vi "Get Cluster Element Names.vi"(8 "error in (no error)":errorcluster, 10 "Cluster":variant) -> (0 "error out":errorcluster, 2 "Element Names":string[](array[string]))   [LabVIEW 2020]
doc: "Returns the data names of the cluster elements."
panel:
  # "[OpenG VI Tags] ***Do Not Remove***"
  # "Get Cluster Element Names.vi\n\nReturns the data names of the cluster elements.\n\nPlease visit http://www.OpenG.org to learn about the\nOpen Source LabVIEW software movement.\n\nNOTICE -- YOU MUST LEAVE THIS NOTICE IN PLACE.  PER THE TERMS OF THE LICENSE BELOW, YOU MAY SUBLICENSE THIS SOFTWARE \nIN ANY WAY THAT DOES NOT CONFLICT WITH THIS LICENSE.\n\n### BSD License (http://www.opensource.org/licenses/bsd-license.php) Begin ###\n \nCopyright (c) 2002, Jean-Pierre Drolet <drolet_jp@hotmail.com>\nCopyright (c) 2002-2006, Jim Kring <jim@jimkring.com>\n\nAll rights reserved.\n\nRedistribution and use in source and binary forms, with or without modification, are permitted provided that the following conditions are met:\n\n    * Redistributions of source code must retain the above copyright notice, this list of conditions and the following disclaimer.\n    * Redistributions in binary form must reproduce the above copyright notice, this list of conditions and the following disclaimer in the \n       documentation and/or other materials provided with the distribution.\n    * Neither the name of SciWare, James Kring, Inc., nor the names of its contributors may be used to endorse or promote products derived \n       from this software without specific prior written permission.\n\nTHIS SOFTWARE IS PROVIDED BY THE COPYRIGHT HOLDERS AND CONTRIBUTORS \"AS IS\" AND ANY EXPRESS OR IMPLIED WARRANTIES, \nINCLUDING, BUT NOT LIMITED TO, THE IMPLIED WARRANTIES OF MERCHANTABILITY AND FITNESS FOR A PARTICULAR PURPOSE ARE \nDISCLAIMED. IN NO EVENT SHALL THE COPYRIGHT OWNER OR CONTRIBUTORS BE LIABLE FOR ANY DIRECT, INDIRECT, INCIDENTAL,\n SPECIAL, EXEMPLARY, OR CONSEQUENTIAL DAMAGES (INCLUDING, BUT NOT LIMITED TO, PROCUREMENT OF SUBSTITUTE GOODS OR \nSERVICES; LOSS OF USE, DATA, OR PROFITS; OR BUSINESS INTERRUPTION) HOWEVER CAUSED AND ON ANY THEORY OF LIABILITY, \nWHETHER IN CONTRACT, STRICT LIABILITY, OR TORT (INCLUDING NEGLIGENCE OR OTHERWISE) ARISING IN ANY WAY OUT OF THE USE \nOF THIS SOFTWARE, EVEN IF ADVISED OF THE POSSIBILITY OF SUCH DAMAGE.\n\n### BSD License End ###"
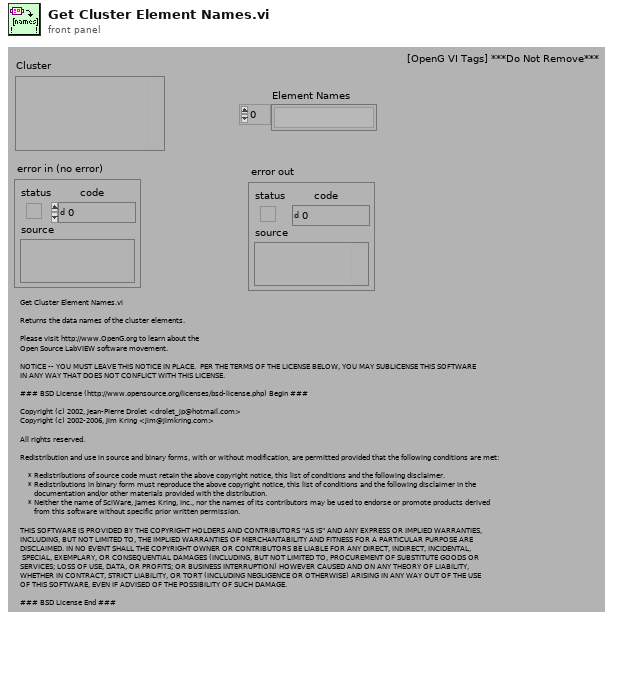
[diagram p1: front panel]
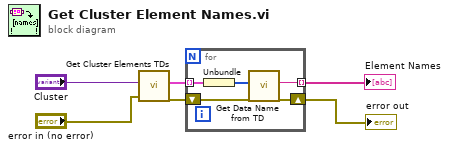
[diagram p0: block diagram]
diagram:
  n1 = call "Get Cluster Elements TDs.vi"("error in (no error)"="error in (no error)", "Cluster"="Cluster") -> ("error out"=w3:errorcluster, "type strings"=w2:cluster{"type string":i16[]}[])  [unwired: 8 in]
  n2 = for {
    tunnel: w2 -> [w8] mode=indexing
    shift-right: [w9] -> w6
    shift-left: w3 -> [w11]
    tunnel: [w10] -> w5 mode=indexing
    n3 = Unbundle(w8) -> ("type string"=w7:i16[])
    n4 = call "Get Data Name from TD.vi"("error in (no error)"=w11, "Type Descriptor"=w7) -> ("error"=w9:errorcluster, "name"=w10:string)  [unwired: 8 in]
  }
  "error out" <- w6
  "Element Names" <- w5
